vi "load_xml.vi"(8 "error in":errorcluster, 10 "child node in":refnum<k20>, 11 "GPIB (in)":refnum<class "GPIB.lvclass">) -> (0 "error out":errorcluster, 2 "child node out":refnum<k20>)   [LabVIEW 2013, in "GPIB.lvclass"]
doc: "Loads analog output settings from xml. Expected format:\n\n<Enable>%b</Enable>\n<PhysicalChannel>%s</PhysicalChannel>\n<MinimumValue>%f</MinimumValue>\n<MaximumValue>%f</MaximumValue>\n<SamplesPerSecond>%f</SamplesPerSecond>\n<TotalAOTime units=\"seconds\">%s</TotalAOTime>\n<AnalogOutputEquations>\n%s</AnalogOutputEquations>\n<StartTrigger.WaitForStartTrigger>%b</StartTrigger.WaitForStartTrigger\n<StartTrigger.source>%s</StartTrigger.source>\n<StartTrigger.edge>%s</StartTrigger.edge>\n\nMTL 2012 Dec 31"
uses:
  GPIB.lvclass
  GPIB.lvclass/GPIB.ctl
  HP83623A_RF_Generator/HP83623A_RF_Generator.lvclass
  HP8662A_RF_Generator/HP8662A_RF_Generator.lvclass
  HP83712B_RF_Generator/HP83712B_RF_Generator.lvclass
  <vilib>/xml/Close Reference(Node).vi
  <resource>/objmgr/DOMUserDefRef.rc
  <vilib>/xml/NI_XML.lvlib
panel:
  out "GPIB":refnum<class "GPIB.lvclass">
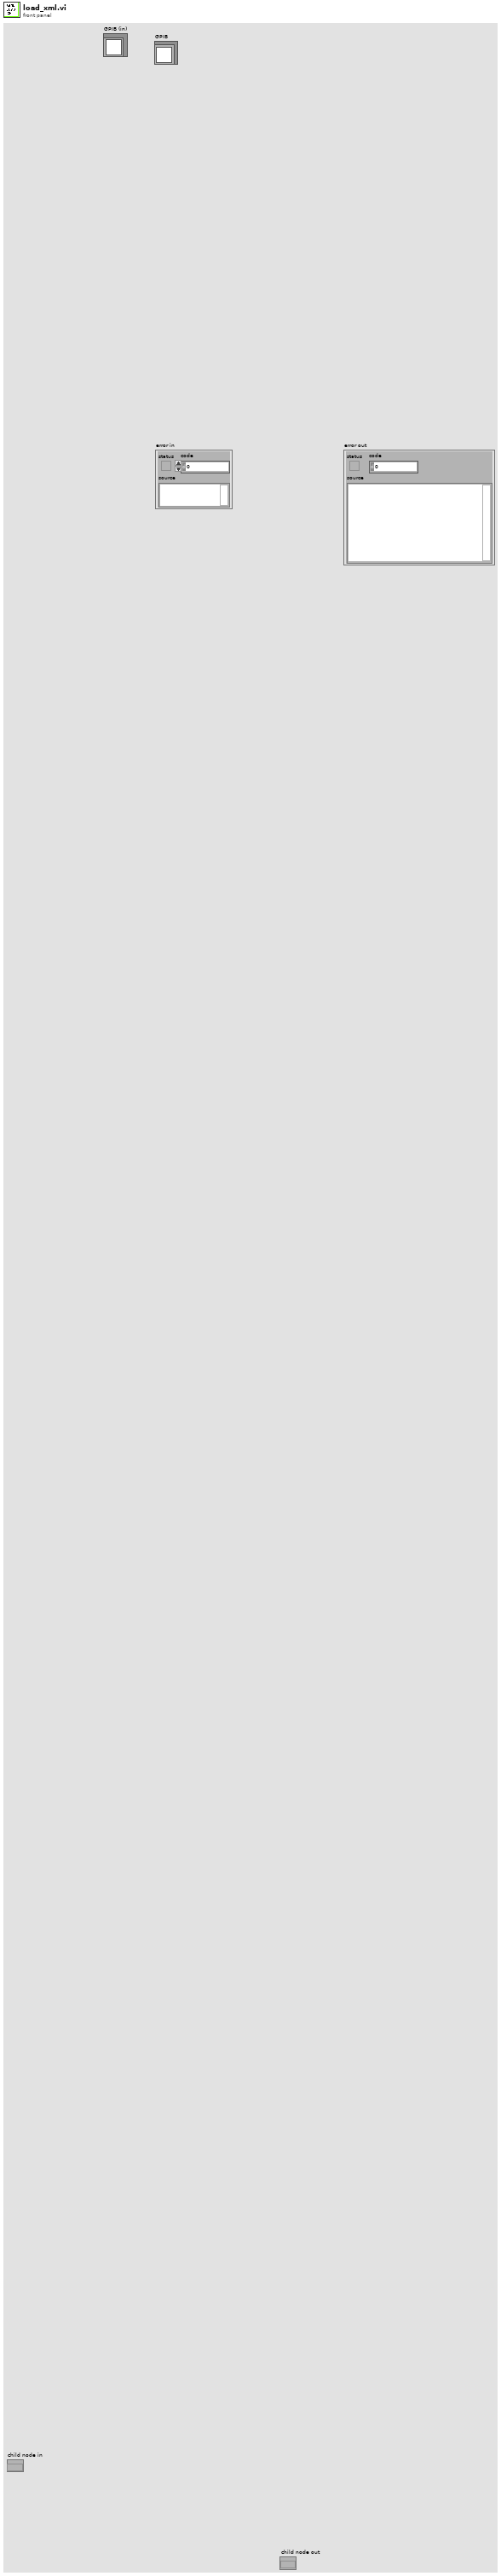
[diagram p1: front panel]
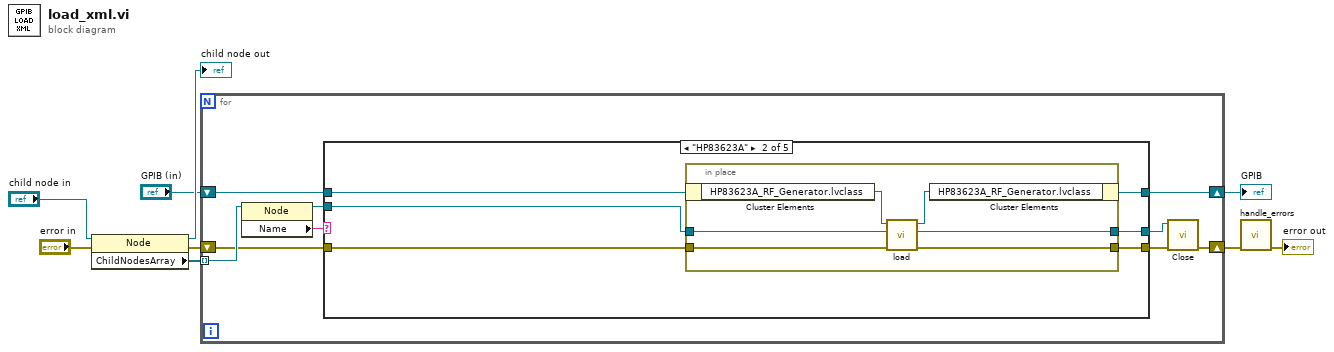
[diagram p0: block diagram]
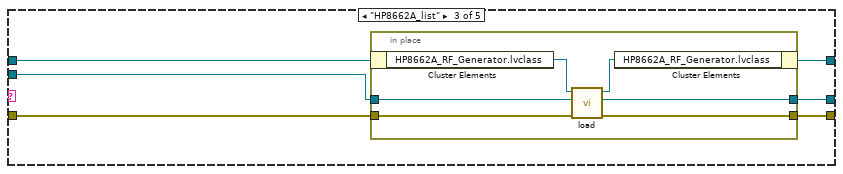
[diagram p3: hidden frame]
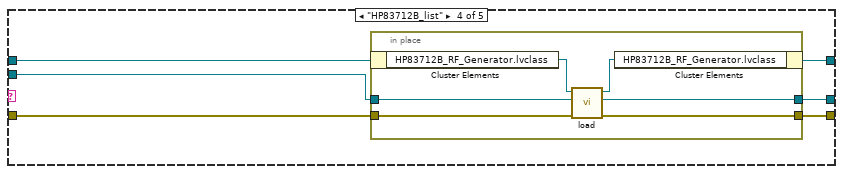
[diagram p4: hidden frame]
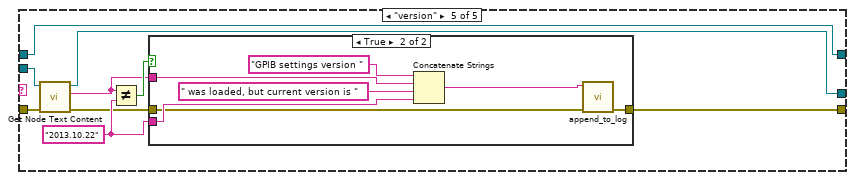
[diagram p5: hidden frame]
diagram:
  n1 = property class="Node"(reference="child node in", error in="error in") -> (reference out=→"child node out":refnum<k20>, error out=w3:errorcluster, "ChildNodesArray"=w4:refnum<k20>[])
  n2 = for {
    tunnel: w4 -> [w18] mode=indexing
    shift-right: [w12] -> w8
    shift-left: w3 -> [w15]
    shift-right: [w10] -> w1
    shift-left: "GPIB (in)" -> [w11]
    n3 = property class="Node"(reference=w18) -> (reference out=w17:refnum<k20>, "Name"=w16:string)  [unwired: 1 in, 1 out]
    n4 = case shown="\"HP83623A\"" w16 {
      tunnel: [w21 w22 w35 w46 w59] -> w14
      tunnel: w17 -> [w21 w25 w38 w49 w62]
      tunnel: w15 -> [w20 w24 w37 w48 w61]
      tunnel: [w20 w23 w36 w47 w60] -> w13
      tunnel: w11 -> [w19 w27 w39 w51 w58]
      tunnel: [w19 w26 w34 w50 w58] -> w10
      frame "None", Default {
      }
      frame "HP83623A" {
        n5 = in-place {
          in-place-border: w25 -> [w33]
          in-place-border: w24 -> [w30]
          in-place-border: [w29] -> w23
          in-place-border: [w28] -> w22
          n6 = in-place-cluster #1(w27) -> ("HP83623A_RF_Generator.lvclass"=w32:refnum<class "HP83623A_RF_Generator.lvclass">)
          n7 = call-dynamic "load.vi"("error in (no error)"=w30, "Node"=w33, "HP83623A_RF_Generator in"=w32) -> ("error out"=w29:errorcluster, "node out"=w28:refnum<k20>, "HP83623A_RF_Generator out"=w31:refnum<class "HP83623A_RF_Generator.lvclass">)  [unwired: 6 in]
          n8 = in-place-cluster #1("HP83623A_RF_Generator.lvclass"=w31) -> (w26:refnum<class "GPIB.lvclass">)
        }
      }
      frame "HP8662A_list" {
        n9 = in-place {
          in-place-border: w38 -> [w43]
          in-place-border: w37 -> [w42]
          in-place-border: [w41] -> w36
          in-place-border: [w40] -> w35
          n10 = in-place-cluster #2(w39) -> ("HP8662A_RF_Generator.lvclass"=w45:refnum<class "HP8662A_RF_Generator.lvclass">)
          n11 = call-dynamic "load.vi"("error in (no error)"=w42, "Node"=w43, "HP8662A_RF_Generator in"=w45) -> ("error out"=w41:errorcluster, "node out"=w40:refnum<k20>, "HP8662A_RF_Generator out"=w44:refnum<class "HP8662A_RF_Generator.lvclass">)  [unwired: 6 in]
          n12 = in-place-cluster #2("HP8662A_RF_Generator.lvclass"=w44) -> (w34:refnum<class "GPIB.lvclass">)
        }
      }
      frame "HP83712B_list" {
        n13 = in-place {
          in-place-border: w49 -> [w57]
          in-place-border: w48 -> [w54]
          in-place-border: [w53] -> w47
          in-place-border: [w52] -> w46
          n14 = in-place-cluster #3(w51) -> ("HP83712B_RF_Generator.lvclass"=w55:refnum<class "HP83712B_RF_Generator.lvclass">)
          n15 = call-dynamic "load.vi"("error in (no error)"=w54, "Node"=w57, "HP83712B_RF_Generator in"=w55) -> ("error out"=w53:errorcluster, "node out"=w52:refnum<k20>, "HP83712B_RF_Generator out"=w56:refnum<class "HP83712B_RF_Generator.lvclass">)  [unwired: 6 in]
          n16 = in-place-cluster #3("HP83712B_RF_Generator.lvclass"=w56) -> (w50:refnum<class "GPIB.lvclass">)
        }
      }
      frame "version" {
        w64 = "2013.10.22" ("y")
        n17 = call <vilib>:"Get Node Text Content.vi"("error in (no error)"=w61, "node in"=w62) -> ("error out"=w63:errorcluster, "node text"=w65:string, "node out"=w59:refnum<k20>)  [unwired: 7 in]
        n18 = Not Equal?(x=w65, y=w64) -> (x != y?=w66:bool)
        n19 = case shown="True" w66 {
          tunnel: w65 -> [_ w73]
          tunnel: w64 -> [_ w71]
          tunnel: w63 -> [w67 w69]
          tunnel: [w67 w68] -> w60
          frame False {
          }
          frame True {
            n20 = Concatenate Strings("GPIB settings version " ("string"), w73, " was loaded, but current version is " ("string"), w71) -> (w70:string)
            n21 = call "append_to_log.vi"("error in"=w69, "string"=w70) -> ("error out"=w68:errorcluster)  [unwired: 9 in]
          }
        }
      }
    }
    n22 = call-poly <vilib>:"Close.vi"("error in (no error)"=w13, "node"=w14) -> ("error out"=w12:errorcluster)  [unwired: 7 in]
  }
  "GPIB" <- w1
  n23 = call "handle_errors.vi"("error in (no error)"=w8) -> ("error out"=→"error out":errorcluster)  [unwired: 10 in]
